vi "AB_850_860_Project_App_Info.vi"(7 "action":T1, 8 "error in (no error)":errorcluster, 9 "buildTypeGUID":string, 10 "applicationInfo in":T2, 11 "Object In":T3) -> (0 "error out":errorcluster, 2 "Application info":T2, 3 "Object Out":T3)   [LabVIEW 2020]
uses:
  <resource>/Framework/Providers/API/ItemRef.ctl
  <vilib>/AppBuilder/RW_Project/AB_RW_Project_PropBag_Action.ctl
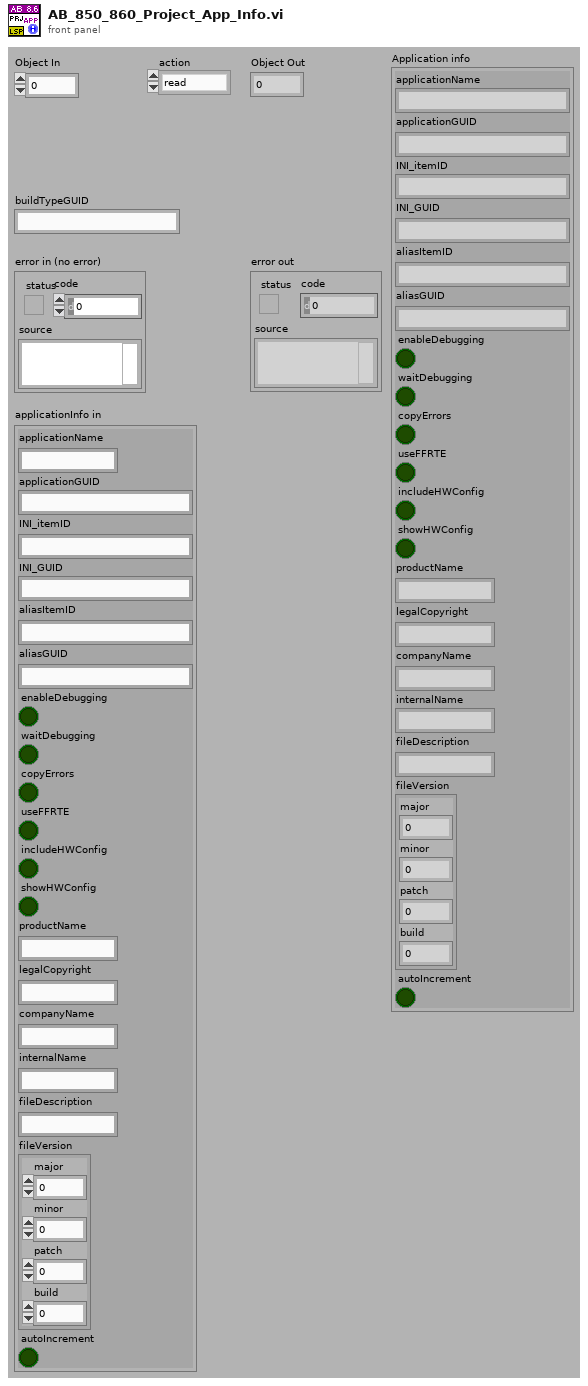
[diagram p1: front panel]
types:
  T1 = typedef "AB_RW_Project_PropBag_Action.ctl" = enum16{"read", "write", "clear", "readPrevious", "writePrevious", "clearPrevious"}
  T2 = cluster{"applicationName":string, "applicationGUID":string, "INI_itemID":string, "INI_GUID":string, "aliasItemID":string, "aliasGUID":string, "enableDebugging":bool, "waitDebugging":bool, "copyErrors":bool, "useFFRTE":bool, "includeHWConfig":bool, "showHWConfig":bool, "productName":string, "legalCopyright":string, "companyName":string, "internalName":string, "fileDescription":string, "fileVersion":cluster{"major":u16, "minor":u16, "patch":u16, "build":u16}, "autoIncrement":bool}
  T3 = typedef "ItemRef.ctl" = u64
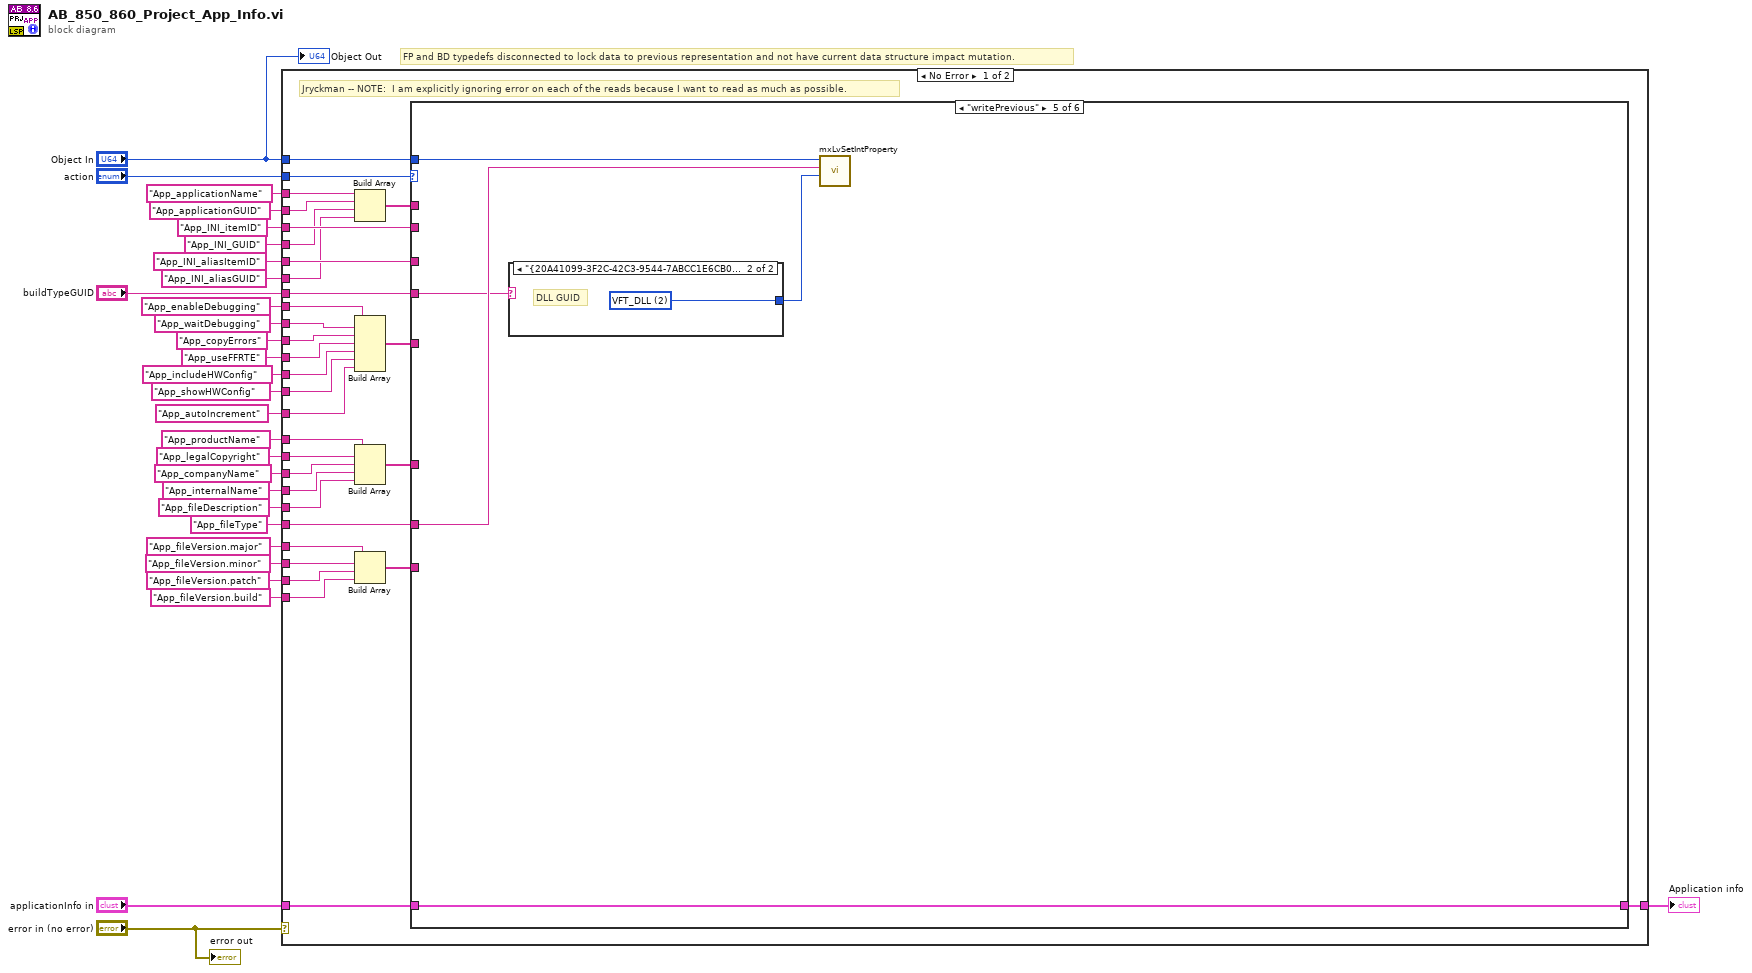
[diagram p0: block diagram]
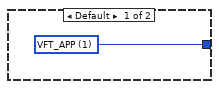
[diagram p6: hidden frame]
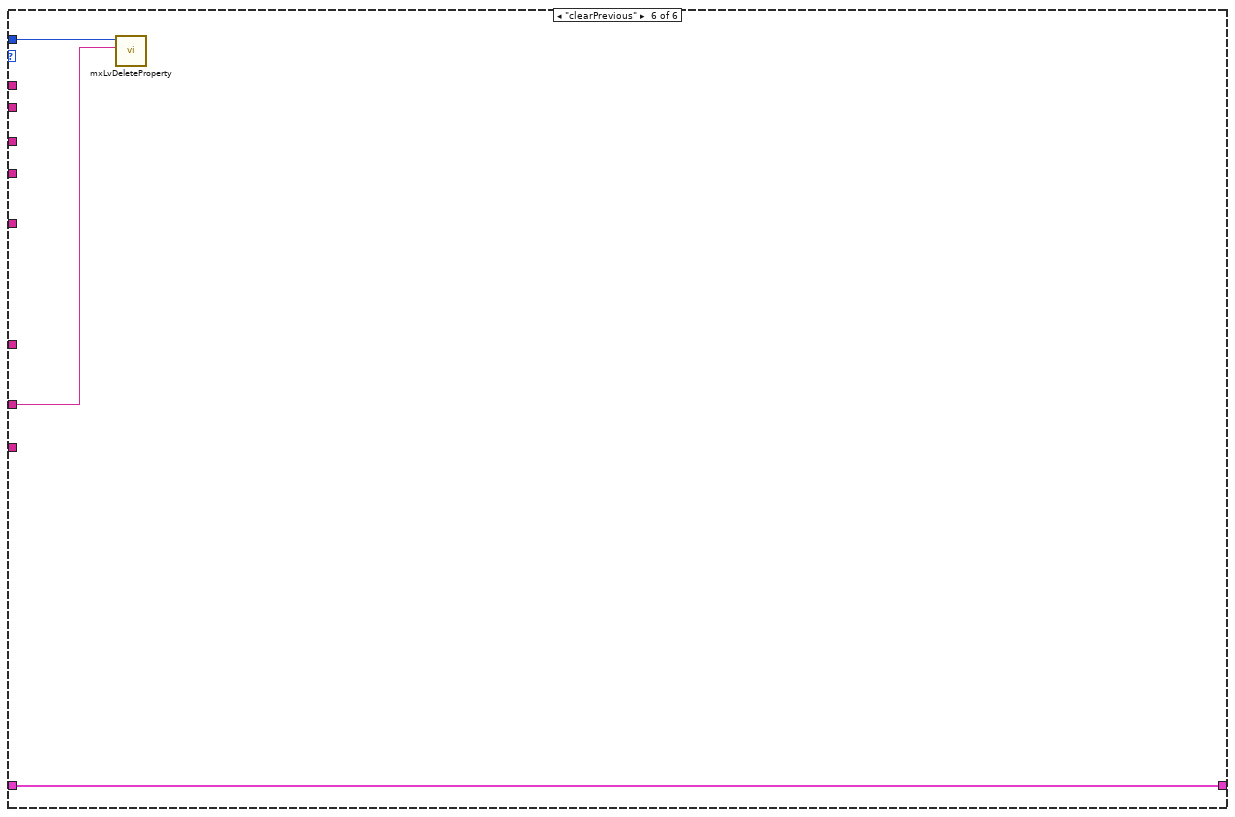
[diagram p7: hidden frame]
diagram:
  # "FP and BD typedefs disconnected to lock data to previous representation and not have current data structure impact mutation."
  n1 = case shown="No Error" "error in (no error)" {
    tunnel: "Object In" -> [w61 _]
    tunnel: [w38 _] -> w27
    tunnel: "applicationInfo in" -> [w44 _]
    tunnel: "App_applicationName" ("Tag") -> [w35 _]
    tunnel: "App_INI_itemID" ("Tag") -> [w60 _]
    tunnel: "App_INI_aliasItemID" ("Tag") -> [w59 _]
    tunnel: "App_enableDebugging" ("Tag") -> [w58 _]
    tunnel: "App_waitDebugging" ("Tag") -> [w57 _]
    tunnel: "App_copyErrors" ("Tag") -> [w56 _]
    tunnel: "App_useFFRTE" ("Tag") -> [w55 _]
    tunnel: "App_includeHWConfig" ("Tag") -> [w54 _]
    tunnel: "App_showHWConfig" ("Tag") -> [w53 _]
    tunnel: "App_productName" ("Tag") -> [w49 _]
    tunnel: "App_legalCopyright" ("Tag") -> [w50 _]
    tunnel: "App_companyName" ("Tag") -> [w48 _]
    tunnel: "App_internalName" ("Tag") -> [w47 _]
    tunnel: "App_fileDescription" ("Tag") -> [w46 _]
    tunnel: "App_fileType" ("Tag") -> [w36 _]
    tunnel: "App_fileVersion.major" ("Tag") -> [w42 _]
    tunnel: "App_fileVersion.minor" ("Tag") -> [w43 _]
    tunnel: "App_fileVersion.patch" ("Tag") -> [w41 _]
    tunnel: "App_fileVersion.build" ("Tag") -> [w40 _]
    tunnel: "App_autoIncrement" ("Tag") -> [w52 _]
    tunnel: "action" -> [w37 _]
    tunnel: "App_applicationGUID" ("Tag") -> [w34 _]
    tunnel: "App_INI_GUID" ("Tag") -> [w33 _]
    tunnel: "App_INI_aliasGUID" ("Tag") -> [w32 _]
    tunnel: "buildTypeGUID" -> [w30 _]
    frame No Error {
      # "Jryckman -- NOTE:  I am explicitly ignoring error on each of the reads because I want to read as much as possible."
      n2 = Build Array(w35, w34, w33, w32) -> (w31:string[])
      n3 = Build Array(w58, w57, w56, w55, w54, w53, w52) -> (w51:string[])
      n4 = Build Array(w49, w50, w48, w47, w46) -> (w45:string[])
      n5 = Build Array(w42, w43, w41, w40) -> (w39:string[])
      n6 = case shown="\"writePrevious\"" w37 {
        tunnel: w61 -> [_ _ _ _ w70 w74]
        tunnel: w60 -> [_ _ _ _ _ _]
        tunnel: w59 -> [_ _ _ _ _ _]
        tunnel: w51 -> [_ _ _ _ _ _]
        tunnel: w45 -> [_ _ _ _ _ _]
        tunnel: w44 -> [w62 w63 w64 w65 w67 w75]
        tunnel: w39 -> [_ _ _ _ _ _]
        tunnel: [w62 w63 w64 w65 w67 w75] -> w38
        tunnel: w36 -> [_ _ _ _ w69 w73]
        tunnel: w31 -> [_ _ _ _ _ _]
        tunnel: w30 -> [_ _ _ _ w68 _]
        frame "read" {
        }
        frame "write" {
        }
        frame "clear" {
        }
        frame "readPrevious" {
        }
        frame "writePrevious" {
          n7 = case shown="\"{20A41099-3F2C-42C3-9544-7ABCC1E6CB0D}\"" w68 {
            tunnel: [w71 w72] -> w66
            frame Default {
              w71 = u16 1 items=["VFT_UNKNOWN", "VFT_APP", "VFT_DLL", "VFT_DRV", "VFT_FONT", "VFT_VXD", "-", "VFT_STATIC_LIB"] ("FileType")
            }
            frame "{20A41099-3F2C-42C3-9544-7ABCC1E6CB0D}" {
              w72 = u16 2 items=["VFT_UNKNOWN", "VFT_APP", "VFT_DLL", "VFT_DRV", "VFT_FONT", "VFT_VXD", "-", "VFT_STATIC_LIB"] ("FileType")
              # "DLL GUID"
            }
          }
          n8 = call <resource>:"mxLvSetIntProperty.vi"("Value (0)"=w66, "Tag"=w69, "Item"=w70) -> ()  [unwired: 2 in, 7 out]
        }
        frame "clearPrevious" {
          n9 = call <resource>:"mxLvDeleteProperty.vi"("Tag"=w73, "Item"=w74) -> ()  [unwired: 1 in, 9 out]
        }
      }
    }
    frame Error {
    }
  }
  "Application info" <- w27
  "Object Out" <- "Object In"
  "error out" <- "error in (no error)"
